vi "Main.vi"() -> ()   [LabVIEW 2021]
uses:
  <vilib>/DAQmx/write.llb/DAQmx Write (Analog DBL 1Chan 1Samp).vi
  <vilib>/DAQmx/read.llb/DAQmx Read (Analog 1D Wfm NChan NSamp).vi
  <vilib>/DAQmx/create/channels.llb/DAQmx Create Channel (AI-Voltage-Basic).vi
  <vilib>/DAQmx/configure/timing.llb/DAQmx Timing (Sample Clock).vi
  <vilib>/DAQmx/create/channels.llb/DAQmx Create Channel (AO-Voltage-Basic).vi
  <vilib>/DAQmx/miscellaneous.llb/DAQmx Fill In Error Info.vi
  <vilib>/Utility/TDMS File Viewer/NI_TDMS File Viewer.lvlib
  <resource>/objmgr/daqmx.rc
panel:
  out "SampClk.Rate":dbl
  out "Waveform Chart":waveform(dbl)[](graph)
  out "Loop":i32
  in  "data":dbl(slide) scale=-10.0..10.0
  out "Elapsed Time":dbl format="%#_6f"
  out "path":path
  in  "stop":bool
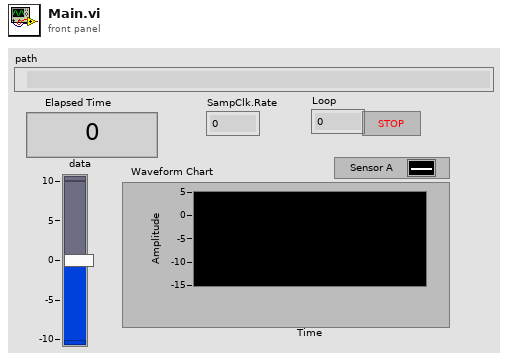
[diagram p1: front panel]
types:
  T1 = enum16{"open", "open or create", "create or replace", "create", "open (read-only)"}
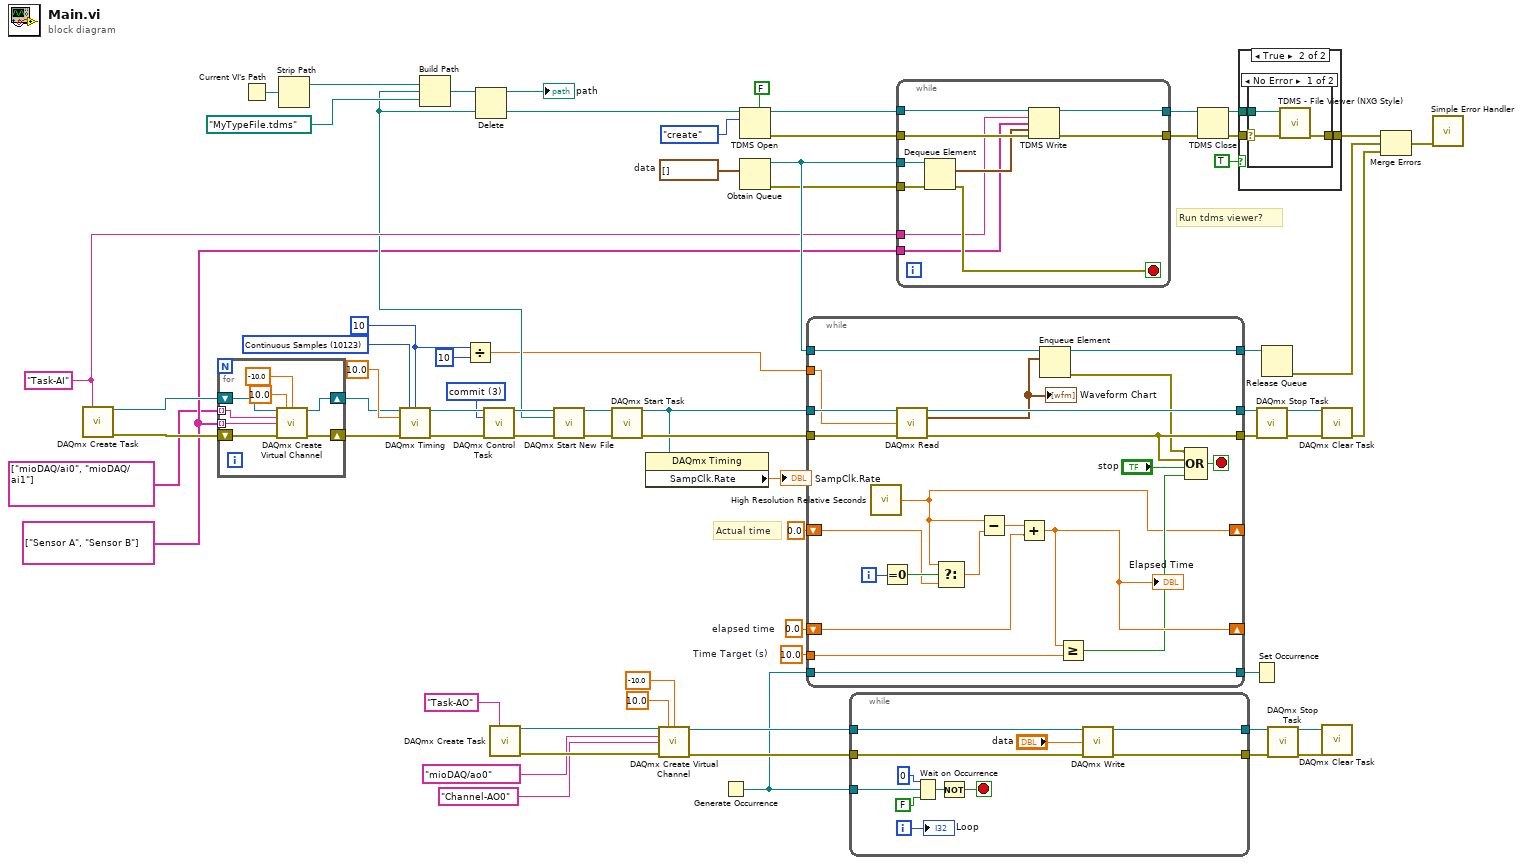
[diagram p0: block diagram]
diagram:
  w17 = waveform(dbl)[] []  # data
  w36 = 10.0  # Time Target (s)
  w37 = 0.0  # elapsed time
  w2 = string[] ["Sensor A", "Sensor B"] ("name to assign")
  w5 = 10 ("samples per channel")
  w40 = 10123 items=["Finite Samples"=10178, "Continuous Samples"=10123, "Hardware Timed Single Point"=12522] ("sample mode")
  w43 = 3 items=["verify"=2, "reserve"=4, "commit"=3, "unreserve"=5, "abort"=6] ("action")
  w38 = "Task-AI" ("new task name")
  # "Run tdms viewer?"
  # "Actual time"
  n1 = call <vilib>:"DAQmx Create Task.vi"("new task name"=w38) -> ("task out"=w56:refnum<k21>, "error out"=w55:errorcluster)  [unwired: 13 in]
  n2 = for {
    shift-right: [w71] -> w9
    shift-left: w56 -> [w73]
    shift-right: [w74] -> w60
    shift-left: w55 -> [w72]
    tunnel: w2 -> [w68] mode=indexing
    tunnel: tag[] ["mioDAQ/ai0", "mioDAQ/ai1"] ("physical channels") -> [w67] mode=indexing
    n3 = call-poly <vilib>:"DAQmx Create Virtual Channel.vi"("task in"=w73, "maximum value"=10.0, "minimum value"=-10.0, "physical channels"=w67, "name to assign"=w68, "error in"=w72) -> ("task out"=w71:refnum<k21>, "error out"=w74:errorcluster)  [unwired: 8 in]
  }
  n4 = Current VI's Path() -> (path=w66:path)
  n5 = Strip Path(path=w66) -> (stripped path=w65:path)  [unwired: 1 out]
  n6 = call-poly <vilib>:"DAQmx Timing.vi"("task/channels in"=w9, "sample mode"=w40, "samples per channel"=w5, "rate"=10.0, "error in"=w60) -> ("task out"=w44:refnum<k21>, "error out"=w45:errorcluster)  [unwired: 9 in]
  n7 = Build Path(base path=w65, name or relative path=path "MyTypeFile.tdms") -> (appended path=w63:path)
  n8 = Divide(x=w5, y=10) -> (x/y=w3:dbl)
  n9 = Delete(path (use dialog)=w63) -> (deleted path=w18:path)  [unwired: 4 in, 2 out]
  "path" <- w18
  n10 = call <vilib>:"DAQmx Control Task.vi"("task/channels in"=w44, "action"=w43, "error in"=w45) -> ("task out"=w42:refnum<k21>, "error out"=w41:errorcluster)  [unwired: 11 in]
  n11 = call <vilib>:"DAQmx Create Task.vi"("new task name"="Task-AO") -> ("task out"=w31:refnum<k21>, "error out"=w30:errorcluster)  [unwired: 13 in]
  n12 = call <vilib>:"DAQmx Start New File.vi"("task/channels in"=w42, "file path"=w18, "error in"=w41) -> ("task out"=w53:refnum<k21>, "error out"=w54:errorcluster)  [unwired: 11 in]
  n13 = call <vilib>:"DAQmx Start Task.vi"("task/channels in"=w53, "error in"=w54) -> ("task out"=w7:refnum<k21>, "error out"=w59:errorcluster)  [unwired: 12 in]
  n14 = property class="DAQmx Timing"(reference=w7) -> ("SampClk.Rate"=→"SampClk.Rate":dbl)  [unwired: 1 in, 2 out]
  n15 = call-poly <vilib>:"DAQmx Create Virtual Channel.vi"("task in"=w31, "maximum value"=10.0, "minimum value"=-10.0, "physical channels"=tag "mioDAQ/ao0", "name to assign"="Channel-AO0", "error in"=w30) -> ("task out"=w29:refnum<k21>, "error out"=w28:errorcluster)  [unwired: 8 in]
  n16 = Generate Occurrence() -> (w19:refnum<k4>)
  n17 = TDMS Open(5:FALSE ("create index file? (T)"), 10:T1."create" ("operation (0:open)"), 11:w18) -> (0:w14:errorcluster, 3:w15:refnum<k34>)  [unwired: 4 in]
  n18 = Obtain Queue(element data type=w17) -> (queue out=w52:refnum<queue>, error out=w16:errorcluster)  [unwired: 4 in, 1 out]
  n19 = while {
    tunnel: w7 -> [w96]
    tunnel: w59 -> [w95]
    tunnel: [w94] -> w58
    tunnel: [w91] -> w57
    tunnel: w52 -> [w93]
    tunnel: [w92] -> w51
    shift-right: [w78] -> _
    shift-left: 0.0 ("relative seconds") -> [w80]
    shift-right: [w86] -> _
    shift-left: w37 -> [w87]
    tunnel: w36 -> [w85]
    tunnel: [w77] -> w20
    tunnel: w19 -> [w77]
    tunnel: w3 -> [w75]
    i -> [w82]
    stop <- w89 stop-if-true
    n20 = call <vilib>:"High Resolution Relative Seconds.vi"() -> ("relative seconds"=w78:dbl)
    n21 = Equal To 0?(x=w82) -> (x = 0?=w81:bool)
    n22 = call-poly <vilib>:"DAQmx Read.vi"("task/channels in"=w96, "number of samples per channel"=w75, "error in"=w95) -> ("task out"=w94:refnum<k21>, "data"=w76:waveform(dbl)[], "error out"=w91:errorcluster)  [unwired: 10 in]
    "Waveform Chart" <- w76
    n23 = Select(t=w78, s=w81, f=w80) -> (s? t:f=w79:dbl)
    n24 = Subtract(x=w78, y=w79) -> (x-y=w88:dbl)
    n25 = Add(x=w88, y=w87) -> (x+y=w86:dbl)
    "Elapsed Time" <- w86
    n26 = Enqueue Element(queue=w93, element=w76) -> (queue out=w92:refnum<queue>, error out=w83:errorcluster)  [unwired: 2 in, 1 out]
    n27 = Greater Or Equal?(x=w86, y=w85) -> (x >= y?=w84:bool)
    n28 = Compound Arithmetic op=OR(w83, w91, "stop", w84) -> (w89:bool)
  }
  n29 = while {
    tunnel: w29 -> [w107]
    tunnel: w28 -> [w106]
    tunnel: [w105] -> w27
    tunnel: [w104] -> w26
    tunnel: w19 -> [w102]
    i -> [w97]
    stop <- w98 stop-if-true
    n30 = Wait on Occurrence(1:FALSE ("ignore previous (T)"), 2:w102, 3:0 ("ms timeout (-1)")) -> (0:w99:bool)
    n31 = Not(x=w99) -> (.not. x?=w98:bool)
    n32 = call-poly <vilib>:"DAQmx Write.vi"("task/channels in"=w107, "data"="data", "error in"=w106) -> ("task out"=w105:refnum<k21>, "error out"=w104:errorcluster)  [unwired: 10 in, 1 out]
    "Loop" <- w97
  }
  n33 = while {
    tunnel: w52 -> [w117]
    tunnel: w16 -> [w115]
    tunnel: w15 -> [w114]
    tunnel: w14 -> [w113]
    tunnel: [w112] -> w50
    tunnel: [w111] -> w49
    tunnel: w2 -> [w108]
    tunnel: w38 -> [w109]
    stop <- w116 stop-if-true
    n34 = Dequeue Element(queue=w117, error in (no error)=w115) -> (element=w110:waveform(dbl)[], error out=w116:errorcluster)  [unwired: 1 in, 2 out]
    n35 = TDMS Write(0:w114, 5:w109, 7:w108, 9:w110, 11:w113) -> (4:w112:refnum<k34>, 15:w111:errorcluster)  [unwired: 1 in, 2 out]
  }
  n36 = TDMS Close(8:w49, 11:w50) -> (0:w11:errorcluster, 3:w10:path)
  n37 = case shown="True" TRUE {
    tunnel: [w118 w121] -> w34
    tunnel: w11 -> [w118 w120]
    tunnel: w10 -> [_ w119]
    frame False {
    }
    frame True {
      n38 = case shown="No Error" w120 {
        selector: w120 -> [w123 w125]
        tunnel: [w124 w125] -> w121
        tunnel: w119 -> [w122 _]
        frame No Error {
          n39 = call <vilib>:"TDMS - File Viewer (NXG Style).vi"("error in"=w123, "file in"=w122) -> ("error out"=w124:errorcluster)  [unwired: 8 in, 1 out]
        }
        frame Error {
        }
      }
    }
  }
  n40 = Set Occurrence(w20) -> ()
  n41 = call <vilib>:"DAQmx Stop Task.vi"("task/channels in"=w58, "error in"=w57) -> ("task out"=w62:refnum<k21>, "error out"=w61:errorcluster)  [unwired: 12 in]
  n42 = Release Queue(queue=w51) -> (error out=w48:errorcluster)  [unwired: 2 in, 2 out]
  n43 = call <vilib>:"DAQmx Stop Task.vi"("task/channels in"=w27, "error in"=w26) -> ("task out"=w33:refnum<k21>, "error out"=w32:errorcluster)  [unwired: 12 in]
  n44 = call <vilib>:"DAQmx Clear Task.vi"("task in"=w62, "error in"=w61) -> ("error out"=w47:errorcluster)  [unwired: 13 in]
  n45 = call <vilib>:"DAQmx Clear Task.vi"("task in"=w33, "error in"=w32) -> ()  [unwired: 13 in, 1 out]
  n46 = Merge Errors(w34, w48, w47) -> (w46:errorcluster)
  n47 = call <vilib>:"Simple Error Handler.vi"("error in (no error)"=w46) -> ()  [unwired: 4 in, 5 out]
